vi "GV-CursorZoomVertStart.vi"(6 "Y":dbl, 7 "Gviewer in":refnum<class "Gviewer.lvclass">, 8 "error in (no error)":errorcluster, 10 "Pos":cluster{"x":i16, "y":i16}, 11 "pict in":picture) -> (0 "error out":errorcluster, 3 "pict out":picture)   [LabVIEW 2020, in "Sgraph_lib_V1.lvlib" / "Gviewer.lvclass"]
doc: "Andre Koelewijn, 8 may 2021\n\nDefine starting point for Vertical Zoom.\nThis function allows zooming for one selected TAG or all TAGs"
uses:
  Gviewer.lvclass
  Gviewer.lvclass/Gviewer.ctl
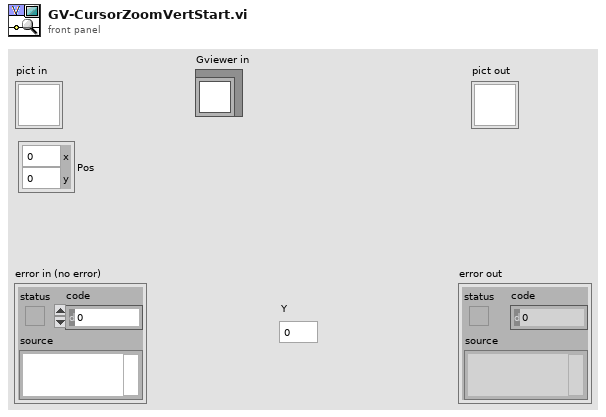
[diagram p1: front panel]
types:
  T1 = cluster{"horizontal":enum16{"left", "center", "right"}, "vertical":enum16{"top", "center", "bottom"}}
  T2 = cluster{"Width":u16, "Style":enum32{"Solid", "Dash", "Dot", "DashDot", "DashDotDot"}}
  T3 = typedef "Sgraph_lib_V1.lvlib/Gviewer.lvclass/Typedef_SelProperties.ctl" = cluster{"Color":u32, "LineType":T4, "max":dbl, "min":dbl}
  T4 = typedef "Sgraph_lib_V1.lvlib/Gviewer.lvclass/Typedef_LineType.ctl" = enum16{"num_bare", "num_MinMax_Area", "num_MinMax_Lines", "num_MinMax_Forfor", "num_Max_Area", "num_Max_Line", "num_Max_Forfor", "num_Min_Area", "num_Min_Line", "num_Min_Fosfor", "Boolean_Line_01", "Boolean_Area_01", "Boolean_Fosfor_01", "Boolean_Line_TF", "Boolean_Area_TF", "Boolean_Fosfor_TF", "Boolean_OnOff_Line", "Boolean_OnOff_Area", "Boolean_OnOff_Fosfor", "Boolean_spare", "StringEvent_Line", "StringEvent_TimeLine"}
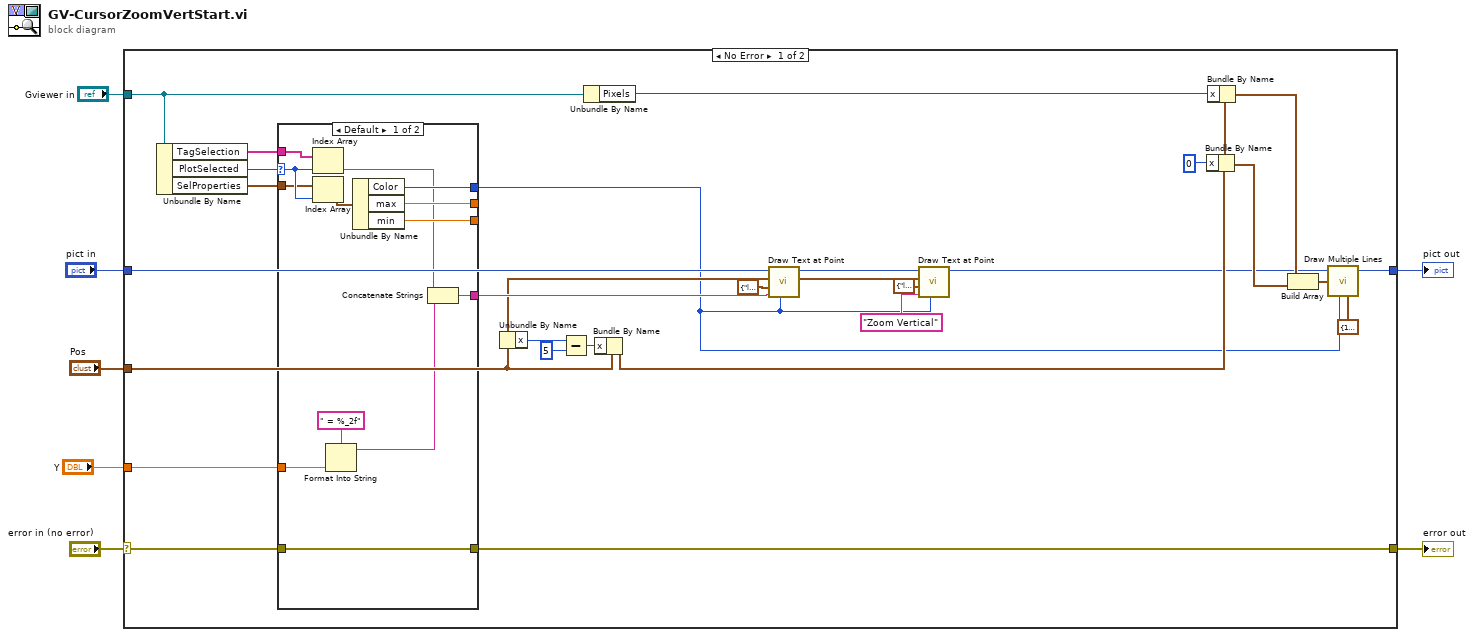
[diagram p0: block diagram]
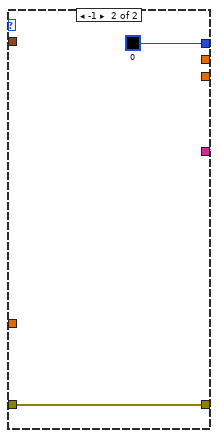
[diagram p2: hidden frame]
diagram:
  n1 = case shown="No Error" "error in (no error)" {
    selector: "error in (no error)" -> [w19 w52]
    tunnel: [w13 w52] -> w6
    tunnel: "pict in" -> [w11 w51]
    tunnel: [w34 w51] -> w4
    tunnel: "Pos" -> [w12 _]
    tunnel: "Gviewer in" -> [w24 _]
    tunnel: "Y" -> [w17 _]
    frame No Error {
      n2 = Unbundle By Name(w24) -> ("TagSelection"=w26:string[], "PlotSelected"=w18:i32, "SelProperties"=w28:T3[])
      n3 = case shown="Default" w18 {
        selector: w18 -> [w44 _]
        tunnel: w26 -> [w47 _]
        tunnel: [w40 "All TAGs"] -> w27
        tunnel: w28 -> [w39 _]
        tunnel: [w45 u32 0 ("Color")] -> w9
        tunnel: [w43 _] -> _
        tunnel: [w42 _] -> _
        tunnel: w19 -> [w36 w48]
        tunnel: [w36 w48] -> w13
        tunnel: w17 -> [w35 _]
        frame Default {
          n4 = Index Array(array=w47, index=w44) -> (element=w41:string)
          n5 = Index Array(array=w39, index=w44) -> (element=w46:T3)
          n6 = Format Into String(format string=" = %_2f", w35) -> (resulting string=w37:string)  [unwired: 2 in, 1 out]
          n7 = Unbundle By Name(w46) -> ("Color"=w45:u32, "max"=w43:dbl, "min"=w42:dbl)
          n8 = Concatenate Strings(w41, w37) -> (w40:string)
        }
        frame -1 {
        }
      }
      n9 = Unbundle By Name(w12) -> ("x"=w22:i16)
      n10 = Subtract(x=w22, y=i16 5) -> (x-y=w20:i16)
      n11 = Unbundle By Name(w24) -> ("Pixels"=w23:i32)
      n12 = Bundle By Name(cluster=w12, "x"=w20) -> (w14:cluster{"x":i16, "y":i16})
      n13 = call <vilib>:"Draw Text at Point.vi"("text color(black)"=w9, "text"=w27, "alignment(left, top)"=T1 {"horizontal"=enum."left", "vertical"=enum."top"}, "origin"=w12, "picture"=w11) -> ("new picture"=w10:picture)  [unwired: 5 in, 1 out]
      n14 = call <vilib>:"Draw Text at Point.vi"("text color(black)"=w9, "text"="Zoom Vertical", "alignment(left, top)"=T1 {"horizontal"=enum."left", "vertical"=enum."bottom"}, "origin"=w12, "picture"=w10) -> ("new picture"=w8:picture)  [unwired: 5 in, 1 out]
      n15 = Bundle By Name(cluster=w14, "x"=i16 0) -> (w32:cluster{"x":i16, "y":i16})
      n16 = Bundle By Name(cluster=w14, "x"=w23) -> (w31:cluster{"x":i16, "y":i16})
      n17 = Build Array(w31, w32) -> (w33:cluster{"x":i16, "y":i16}[])
      n18 = call <vilib>:"Draw Multiple Lines.vi"("picture"=w8, "line endpoints"=w33, "color(black)"=w9, "pen"=T2 {"Width"=1, "Style"=enum."Dot"}) -> ("new picture"=w34:picture)  [unwired: 5 in]
    }
    frame Error {
    }
  }
  "error out" <- w6
  "pict out" <- w4
